vi "Init Module.vi"(8 "error in (no error)":errorcluster, 11 "Event Reporter Module in":refnum<class "Event Reporter Module.lvclass">) -> (0 "error out":errorcluster, 3 "Event Reporter Module out":refnum<class "Event Reporter Module.lvclass">)   [LabVIEW 2020, in "Volatus.lvlib" / "Event Reporter Module.lvclass"]
uses:
  Event Reporter Module.lvclass
  Event Reporter Module.lvclass/Event Reporter Module.ctl
  Event Level.ctl
  Volatus.lvlib
  Event.ctl
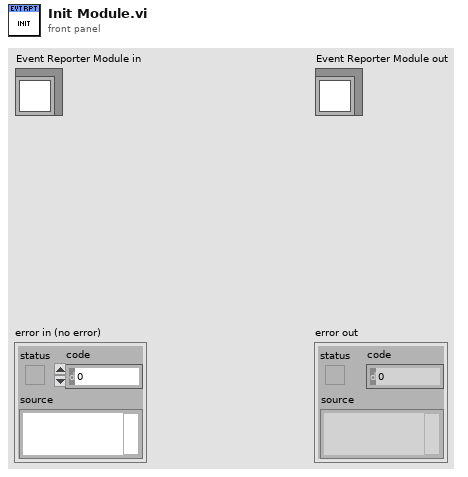
[diagram p1: front panel]
types:
  T1 = typedef "Volatus.lvlib/Event.ctl" = cluster{"Time Stamp":timestamp, "Event Level":T2, "Context":string, "Message":string, "Error":errorcluster}
  T2 = typedef "Volatus.lvlib/Event Level.ctl" = enum16{"Debug", "Info", "Warning", "Error"}
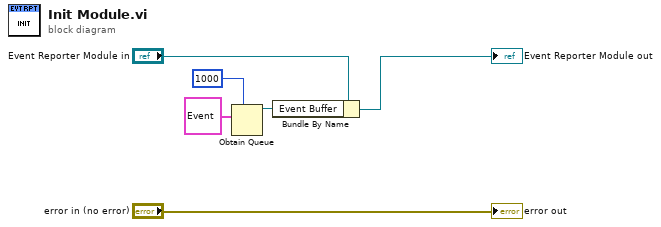
[diagram p0: block diagram]
diagram:
  n1 = Obtain Queue(max queue size (-1, unlimited)=1000, element data type=T1 {"Time Stamp"=timestamp(0 s since 1904-01-01), "Event Level"=enum."Info", "Context"="", "Message"="", "Error"={"status"=FALSE, "code"=0, "source"=""}} ("Event")) -> (queue out=w1:refnum<queue>)  [unwired: 3 in, 2 out]
  n2 = Bundle By Name(cluster="Event Reporter Module in", "Event Buffer"=w1) -> (→"Event Reporter Module out":refnum<class "Event Reporter Module.lvclass">)
  "error out" <- "error in (no error)"
